vi "Get Acquired Data.vi"(8 "error in (no error)":errorcluster, 11 "CCDCamera in":refnum<class "Sim_Ixon_Ultra.lvclass">) -> (0 "error out":errorcluster, 3 "CCDCamera out":refnum<class "Sim_Ixon_Ultra.lvclass">)   [LabVIEW 2018, in "Sim_Ixon_Ultra.lvclass"]
doc: "Get the data acquired by the camera"
uses:
  Sim_Ixon_Ultra.lvclass
  Sim_Ixon_Ultra.lvclass/Sim_Ixon_Ultra.ctl
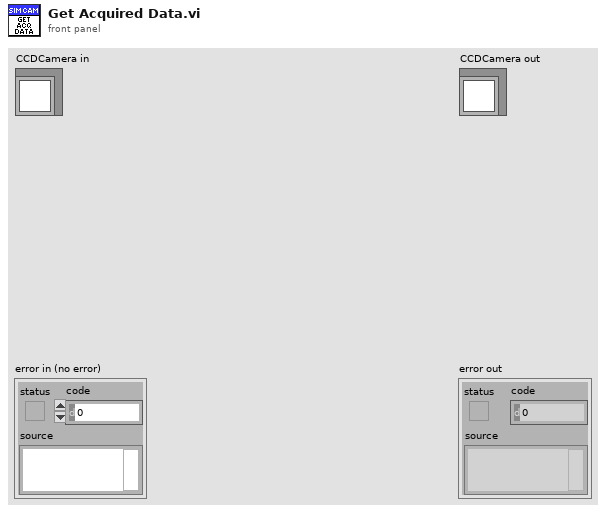
[diagram p1: front panel]
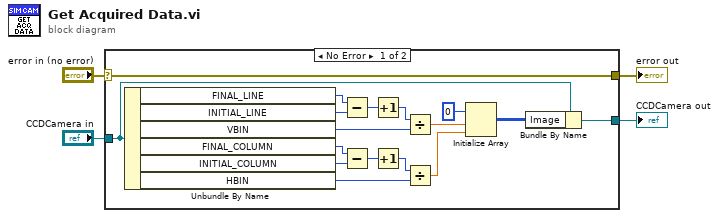
[diagram p0: block diagram]
diagram:
  n1 = case shown="No Error" "error in (no error)" {
    selector: "error in (no error)" -> [w11 w23]
    tunnel: [w11 w23] -> w1
    tunnel: [w21 w22] -> w2
    tunnel: "CCDCamera in" -> [w12 w22]
    frame No Error {
      n2 = Unbundle By Name(w12) -> ("FINAL_LINE"=w10:u16, "INITIAL_LINE"=w9:u16, "VBIN"=w8:u16, "FINAL_COLUMN"=w7:u16, "INITIAL_COLUMN"=w6:u16, "HBIN"=w5:u16)
      n3 = Subtract(x=w10, y=w9) -> (x-y=w20:u16)
      n4 = Subtract(x=w7, y=w6) -> (x-y=w19:u16)
      n5 = Increment(x=w20) -> (x+1=w18:u16)
      n6 = Increment(x=w19) -> (x+1=w17:u16)
      n7 = Divide(x=w18, y=w8) -> (x/y=w15:dbl)
      n8 = Divide(x=w17, y=w5) -> (x/y=w14:dbl)
      n9 = Initialize Array(u16 0, w15, w14) -> (w13:u16[][])
      n10 = Bundle By Name(cluster=w12, "Image"=w13) -> (w21:refnum<class "Sim_Ixon_Ultra.lvclass">)
    }
    frame Error {
    }
  }
  "error out" <- w1
  "CCDCamera out" <- w2
